vi "Guess Module Name.vi"() -> (0 "module name":string)   [LabVIEW 2020, in "MacroAssert.lvlib" / "Winevent.lvlib"]
doc: "This VI attempts to guess whether you are running in the LabVIEW development system or in an executable. To determine this, the VI assumes that it is contained in the .exe."
uses:
  Winevent.lvlib
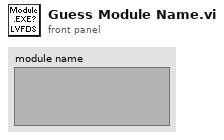
[diagram p1: front panel]
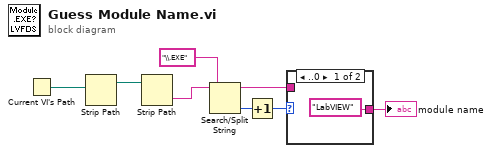
[diagram p0: block diagram]
diagram:
  n1 = Current VI's Path() -> (path=w8:path)
  n2 = Strip Path(path=w8) -> (stripped path=w7:path)  [unwired: 1 out]
  n3 = Strip Path(path=w7) -> (name=w6:string)  [unwired: 1 out]
  n4 = Search/Split String(string=w6, search string/char (-)="\\.EXE") -> (substring before match=w2:string, offset of match=w4:i32)  [unwired: 2 out]
  n5 = Increment(x=w4) -> (x+1=w3:i32)
  n6 = case shown="..0" w3 {
    tunnel: w2 -> [_ w10]
    tunnel: ["LabVIEW" w10] -> w1
    frame ..0 {
    }
    frame 1.. {
    }
  }
  "module name" <- w1
